vi "Save Analysis Results.vi"(0 "VISA resource name":refnum<visa-resource-name>, 1 "Include Mask Statistics (F: Disable)":bool, 2 "Include Search Event Times (F: Disable)":bool, 5 "Output File ()":string, 7 "Include Cursor Values (F: Disable)":bool, 9 "Include Measurement Results (F: Disable)":bool, 11 "error in (no error)":errorcluster, 12 "Include Segmented Memory Acquisition Times (F: Disable)":bool) -> (4 "VISA resource name out":refnum<visa-resource-name>, 15 "error out":errorcluster)   [LabVIEW 2023, in "Keysight-DSQx3014T.lvlib"]
doc: "Saves analysis results to a comma-separated values (*.csv) file on a USB storage device.\nWhen multiple types of analysis results are selected, they are all saved to the same\nfile and separated by a blank line."
uses:
  Keysight-DSQx3014T.lvlib
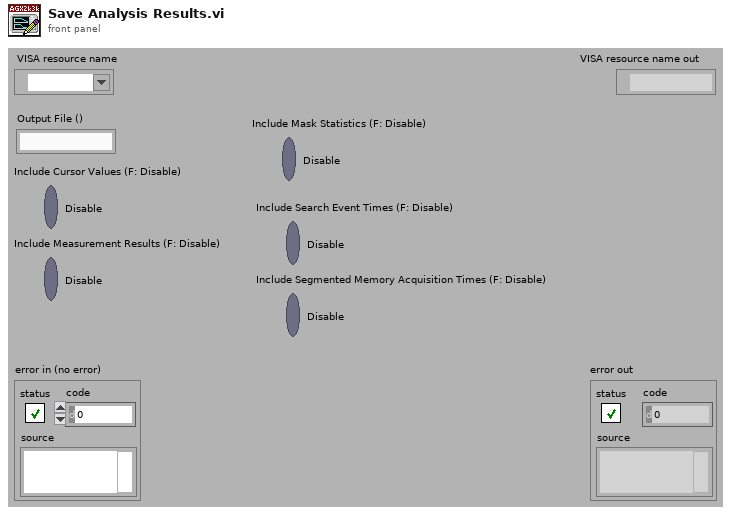
[diagram p1: front panel]
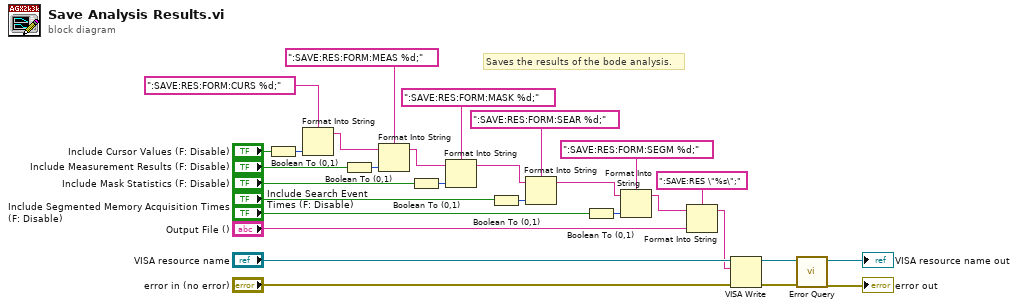
[diagram p0: block diagram]
diagram:
  # "Saves the results of the bode analysis."
  n1 = Boolean To (0,1)(Boolean="Include Cursor Values (F: Disable)") -> (0, 1=w23:i16)
  n2 = Format Into String(format string=":SAVE:RES:FORM:CURS %d;", w23) -> (resulting string=w9:string)  [unwired: 2 in, 1 out]
  n3 = Boolean To (0,1)(Boolean="Include Measurement Results (F: Disable)") -> (0, 1=w19:i16)
  n4 = Format Into String(format string=":SAVE:RES:FORM:MEAS %d;", initial string=w9, w19) -> (resulting string=w10:string)  [unwired: 1 in, 1 out]
  n5 = Boolean To (0,1)(Boolean="Include Mask Statistics (F: Disable)") -> (0, 1=w17:i16)
  n6 = Format Into String(format string=":SAVE:RES:FORM:MASK %d;", initial string=w10, w17) -> (resulting string=w11:string)  [unwired: 1 in, 1 out]
  n7 = Boolean To (0,1)(Boolean="Include Search Event Times (F: Disable)") -> (0, 1=w13:i16)
  n8 = Format Into String(format string=":SAVE:RES:FORM:SEAR %d;", initial string=w11, w13) -> (resulting string=w5:string)  [unwired: 1 in, 1 out]
  n9 = Boolean To (0,1)(Boolean="Include Segmented Memory Acquisition Times (F: Disable)") -> (0, 1=w8:i16)
  n10 = Format Into String(format string=":SAVE:RES:FORM:SEGM %d;", initial string=w5, w8) -> (resulting string=w4:string)  [unwired: 1 in, 1 out]
  n11 = Format Into String(format string=":SAVE:RES \"%s\";", initial string=w4, "Output File ()") -> (resulting string=w1:string)  [unwired: 1 in, 1 out]
  n12 = VISA Write(VISA resource name="VISA resource name", write buffer=w1, error in (no error)="error in (no error)") -> (VISA resource name out=w27:refnum<visa-resource-name>, error out=w26:errorcluster)  [unwired: 1 out]
  n13 = call "Error Query.vi"("error in (no error)"=w26, "VISA resource name"=w27) -> ("error out"=→"error out":errorcluster, "VISA resource name out"=→"VISA resource name out":refnum<visa-resource-name>)  [unwired: 8 out]
